vi "Spectrum Measure.vi"(0 "RFmx Handle In":refnum<k21>, 1 "Selector String":string, 11 "error in (no error)":errorcluster) -> (4 "RFmx Handle Out":refnum<k21>, 6 "Spectrum Results":T1 {"Spectrum"."y" min=0 max=127 format="%.2f"; "Spectrum"."dx" format="%^.2e"; "Spectrum"."x0" format="%^.2e"}, 15 "error out":errorcluster)   [LabVIEW 2018, in "RFmxSpecAn.lvlib"]
uses:
  RFmxSpecAn.lvlib
  Typedefs/Spectrum Results.ctl
  <vilib>/RFmx/SpecAn/mx/RFmxSpecAn.llb/RFmxSpecAn Select Measurement (Single).vi
  <vilib>/RFmx/SpecAn/mx/RFmxSpecAn.llb/RFmxSpecAn Spectrum Fetch Spectrum.vi
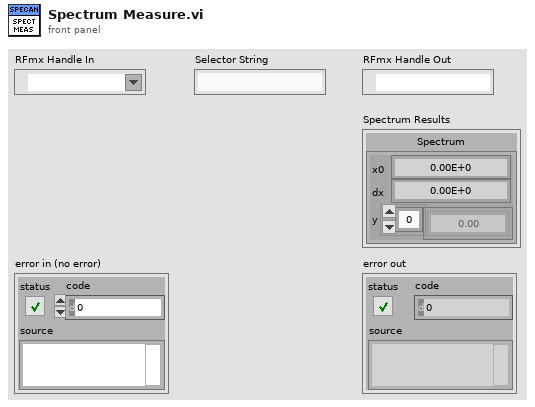
[diagram p1: front panel]
types:
  T1 = typedef "RFmxSpecAn.lvlib/Spectrum Results.ctl" = cluster{"Spectrum":cluster{"x0":dbl, "dx":dbl, "y":sgl[]}}
  T2 = enum16{"ACP", "CCDF", "CHP", "FCnt", "Harmonics", "OBW", "SEM", "Spectrum", "Spur", "TXP", "AMPM", "DPD", "IQ", "IM", "NF", "PhaseNoise"}
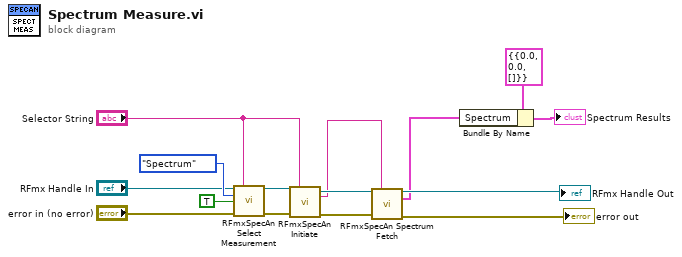
[diagram p0: block diagram]
diagram:
  n1 = call-poly <vilib>:"RFmxSpecAn Select Measurement.vi"("Instrument Handle In"="RFmx Handle In", "Selector String"="Selector String", "Measurement"=T2."Spectrum", "Enable All Traces"=TRUE, "error in (no error)"="error in (no error)") -> ("Instrument Handle Out"=w11:refnum<k21>, "error out"=w10:errorcluster)  [unwired: 9 in]
  n2 = call <vilib>:"RFmxSpecAn Initiate.vi"("Instrument Handle In"=w11, "Selector String"="Selector String", "error in (no error)"=w10) -> ("Instrument Handle Out"=w7:refnum<k21>, "Selector String Out"=w4:string, "error out"=w8:errorcluster)  [unwired: 10 in]
  n3 = call-poly <vilib>:"RFmxSpecAn Spectrum Fetch.vi"("Instrument Handle In"=w7, "Selector String"=w4, "error in (no error)"=w8) -> ("Instrument Handle Out"=→"RFmx Handle Out":refnum<k21>, "Spectrum"=w2:cluster{"x0":dbl, "dx":dbl, "y":sgl[]}, "error out"=→"error out":errorcluster)  [unwired: 10 in]
  n4 = Bundle By Name(cluster=T1 {"Spectrum"={"x0"=0.0, "dx"=0.0, "y"=[]}} ("Spectrum Results"), "Spectrum"=w2) -> (→"Spectrum Results":T1)
